vi "Test Door API.vi"() -> ()   [LabVIEW 2018]
uses:
  Door.lvclass
panel:
  out "error out":errorcluster
  in  "Close Door":bool
  in  "Open Door":bool
  out "Door":u16(ring)
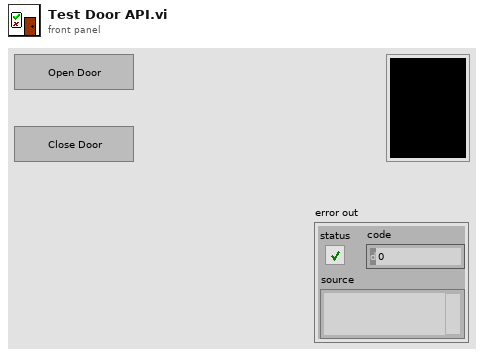
[diagram p1: front panel]
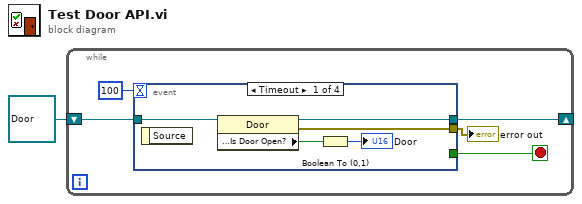
[diagram p0: block diagram]
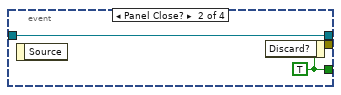
[diagram p2: hidden frame]
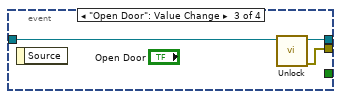
[diagram p3: hidden frame]
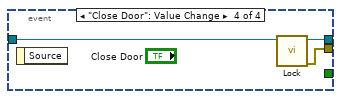
[diagram p4: hidden frame]
diagram:
  n1 = while {
    shift-right: [w3] -> _
    shift-left: refnum<class "Door.lvclass"> refnum ("Door.lvclass") -> [w5]
    stop <- w4 stop-if-true
    n2 = event shown="[0] Timeout" {
      selector: _ -> [_ _ _ _]
      dyn-events: _ -> [_ _ _ _]
      timeout: 100 -> [_ _ _ _]
      tunnel: w5 -> [w11 w12 w16 w19]
      tunnel: [_ w13 _ _] -> w4
      tunnel: [w8 w12 w15 w18] -> w3
      tunnel: [w7 _ w14 w17] -> w2
      event Timeout {
        n3 = event-data() -> ()  [unwired: 1 in, 1 out]
        n4 = property class="Door"(reference=w11) -> (reference out=w8:refnum<class "Door.lvclass">, error out=w7:errorcluster, "Accessors:Is Door Open?"=w10:bool)  [unwired: 1 in]
        n5 = Boolean To (0,1)(Boolean=w10) -> (0, 1=→"Door":i16)
      }
      event Panel Close? {
        w13 = TRUE ("Discard?")
        n6 = event-data() -> ()  [unwired: 1 in, 1 out]
        n7 = event-data("Discard?"=w13) -> ()  [unwired: 1 in, 1 out]
      }
      event "Open Door": Value Change {
        n8 = event-data() -> ()  [unwired: 1 in, 1 out]
        n9 = call-dynamic "Unlock.vi"("Door in"=w16) -> ("error out"=w14:errorcluster, "Door out"=w15:refnum<class "Door.lvclass">)  [unwired: 9 in]
      }
      event "Close Door": Value Change {
        n10 = event-data() -> ()  [unwired: 1 in, 1 out]
        n11 = call-dynamic "Lock.vi"("Door in"=w19) -> ("error out"=w17:errorcluster, "Door out"=w18:refnum<class "Door.lvclass">)  [unwired: 9 in]
      }
    }
    "error out" <- w2
  }
